vi "DataDecode.vi"(5 "Input: lenght":i32=1, 6 "Input: offset":i32, 7 "Input: Data string":string) -> (3 "Output: Decoded Data":i32)   [LabVIEW 2012, in "Serial Controller.lvclass"]
uses:
  Serial Controller.lvclass
panel:
  out "Test: Decoding string (hex)":string
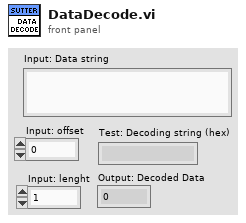
[diagram p1: front panel]
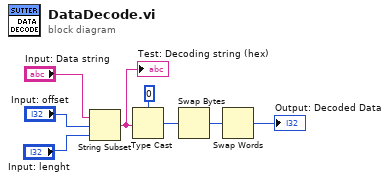
[diagram p0: block diagram]
diagram:
  n1 = String Subset(string="Input: Data string", offset (0)="Input: offset", length (rest)="Input: lenght") -> (substring=w8:string)
  "Test: Decoding string (hex)" <- w8
  n2 = Type Cast(type=0, x=w8) -> (*(type *) &x=w2:i32)
  n3 = Swap Bytes(anything=w2) -> (byte swapped=w1:i32)
  n4 = Swap Words(1:w1) -> (0:→"Output: Decoded Data":i32)
